vi "Read Parameters from First Call.vi"(8 "error in (no error)":errorcluster, 11 "LabSpy in":refnum<class "LabSpy.lvclass">) -> (0 "error out":errorcluster, 2 "First Call Parameters":variant, 3 "LabSpy out":refnum<class "LabSpy.lvclass">)   [LabVIEW 2013, in "LabSpy.lvclass"]
doc: "Get the parameters from the first call of the spy."
uses:
  LabSpy.lvclass
  LabSpy.lvclass/LabSpy.ctl
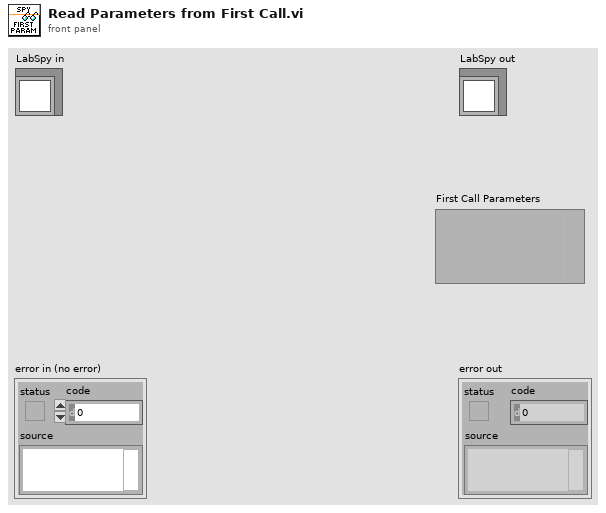
[diagram p1: front panel]
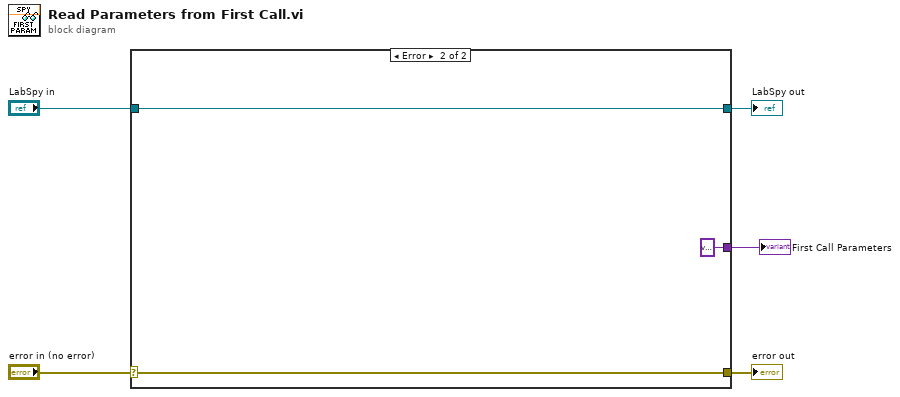
[diagram p0: block diagram]
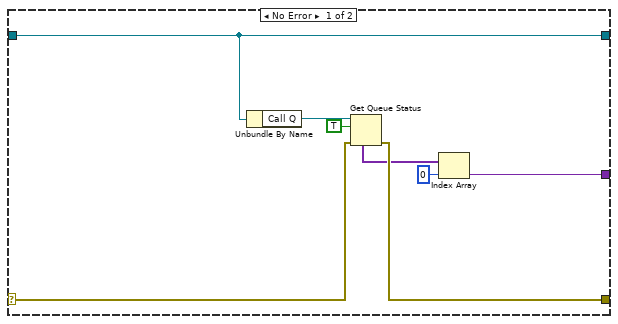
[diagram p2: hidden frame]
diagram:
  n1 = case shown="Error" "error in (no error)" {
    selector: "error in (no error)" -> [w11 w16]
    tunnel: [w10 w16] -> w4
    tunnel: [w13 w15] -> w2
    tunnel: "LabSpy in" -> [w13 w15]
    tunnel: [w6 variant ("Variant")] -> w1
    frame No Error {
      n2 = Unbundle By Name(w13) -> ("Call Q"=w12:refnum<queue>)
      n3 = Get Queue Status(queue=w12, return elements? (F)=TRUE, error in (no error)=w11) -> (error out=w10:errorcluster, elements=w8:variant[])  [unwired: 6 out]
      n4 = Index Array(array=w8, index=0) -> (element=w6:variant)
    }
    frame Error {
    }
  }
  "error out" <- w4
  "LabSpy out" <- w2
  "First Call Parameters" <- w1
